vi "Testing position.vi"(8 "Matched corners":cluster{"X":dbl, "Y":dbl}[](array[cluster]), 11 "Original Found Corners":cluster{"X":dbl, "Y":dbl}[](array[cluster])) -> (3 "Final position":cluster{"X":dbl, "Y":dbl})   [LabVIEW 2016]
panel:
  out "Array":dbl[](array[numeric])
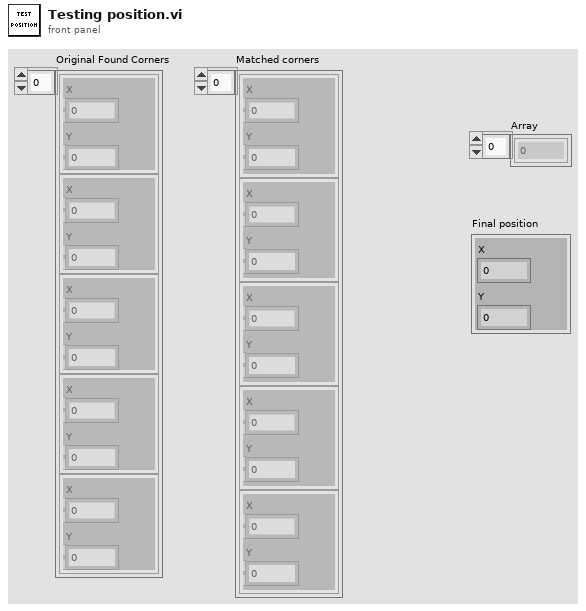
[diagram p1: front panel]
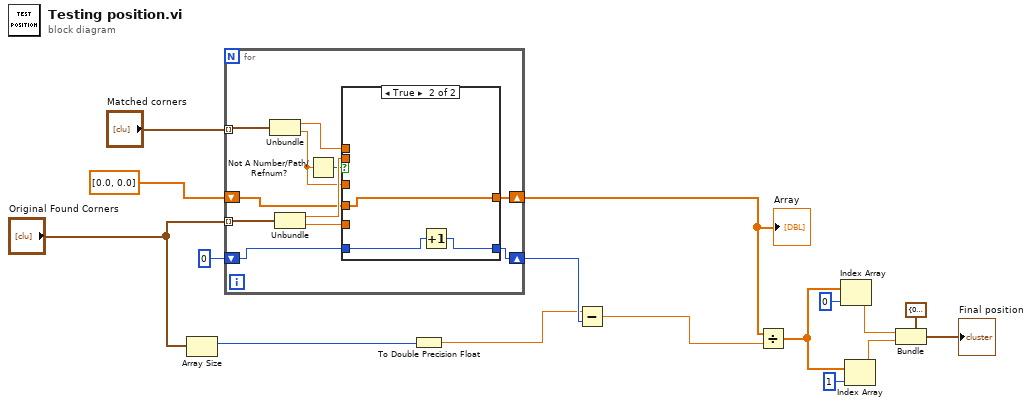
[diagram p0: block diagram]
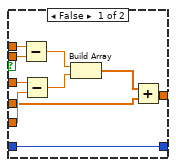
[diagram p2: hidden frame]
diagram:
  n1 = Array Size(array="Original Found Corners") -> (size(s)=w13:i32)
  n2 = for {
    tunnel: "Matched corners" -> [w26] mode=indexing
    tunnel: "Original Found Corners" -> [w27] mode=indexing
    shift-right: [w22] -> w14
    shift-left: dbl[] [0.0, 0.0] -> [w21]
    shift-right: [w17] -> w5
    shift-left: 0 -> [w18]
    n3 = Unbundle(w26) -> ("X"=w25:dbl, "Y"=w19:dbl)
    n4 = Unbundle(w27) -> ("X"=w23:dbl, "Y"=w24:dbl)
    n5 = Not A Number/Path/Refnum?(number/path/refnum=w19) -> (NaN/Path/Refnum?=w20:bool)
    n6 = case shown="True" w20 {
      tunnel: w19 -> [w37 _]
      tunnel: w25 -> [w36 _]
      tunnel: w24 -> [w35 _]
      tunnel: w23 -> [w34 _]
      tunnel: [w30 w40] -> w22
      tunnel: w21 -> [w29 w40]
      tunnel: w18 -> [w28 w38]
      tunnel: [w28 w39] -> w17
      frame False {
        n7 = Subtract(x=w36, y=w34) -> (x-y=w33:dbl)
        n8 = Subtract(x=w37, y=w35) -> (x-y=w32:dbl)
        n9 = Build Array(w33, w32) -> (w31:dbl[])
        n10 = Add(x=w31, y=w29) -> (x+y=w30:dbl[])
      }
      frame True {
        n11 = Increment(x=w38) -> (x+1=w39:i32)
      }
    }
  }
  "Array" <- w14
  n12 = To Double Precision Float(number=w13) -> (double precision float=w4:dbl)
  n13 = Subtract(x=w4, y=w5) -> (x-y=w3:dbl)
  n14 = Divide(x=w14, y=w3) -> (x/y=w11:dbl[])
  n15 = Index Array(array=w11, index=0) -> (element=w9:dbl)
  n16 = Index Array(array=w11, index=1) -> (element=w10:dbl)
  n17 = Bundle(cluster=cluster{"X":dbl, "Y":dbl} {"X"=0.0, "Y"=0.0} ("Final position"), "X"=w9, "Y"=w10) -> (→"Final position":cluster{"X":dbl, "Y":dbl})
